vi "run_chatcompletion_core.vi"(0 "chatcompletion_llm_interface in":refnum<class "abstract_llm_chatcompletion.lvclass">, 5 "Messages":refnum<class "abstract_message_base.lvclass">[](array[class]), 11 "error in (no error)":errorcluster) -> (4 "chatcompletion_llm_interface out":refnum<class "abstract_llm_chatcompletion.lvclass">, 6 "Response":refnum<class "abstract_message_base.lvclass">, 15 "error out":errorcluster)   [LabVIEW 2020, in "abstract_llm_chatcompletion.lvclass"]
uses:
  abstract_llm_chatcompletion.lvclass
  abstract_message_base/abstract_message_base.lvclass
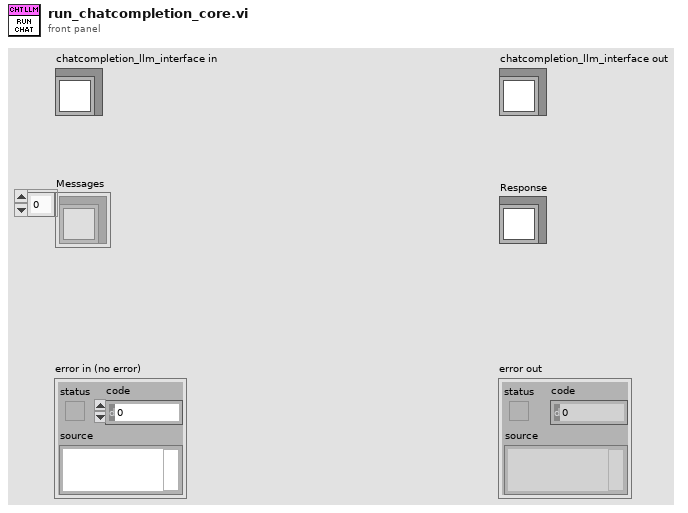
[diagram p1: front panel]
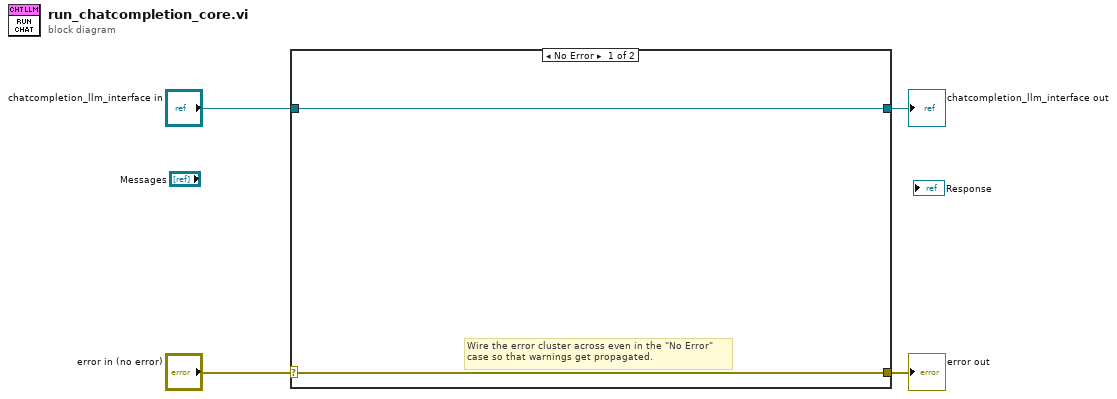
[diagram p0: block diagram]
diagram:
  n1 = case shown="No Error" "error in (no error)" {
    selector: "error in (no error)" -> [w5 w8]
    tunnel: [w5 w8] -> w3
    tunnel: [w6 w7] -> w1
    tunnel: "chatcompletion_llm_interface in" -> [w6 w7]
    frame No Error {
      # "Wire the error cluster across even in the \"No Error\"\ncase so that warnings get propagated."
    }
    frame Error {
    }
  }
  "error out" <- w3
  "chatcompletion_llm_interface out" <- w1
